vi "Close.vi"(8 "error in (no error)":errorcluster, 11 "HD44780 in":refnum<class "HD44780.lvclass">) -> (0 "error out":errorcluster)   [LabVIEW 2017, in "HD44780.lvclass"]
uses:
  HD44780.lvclass
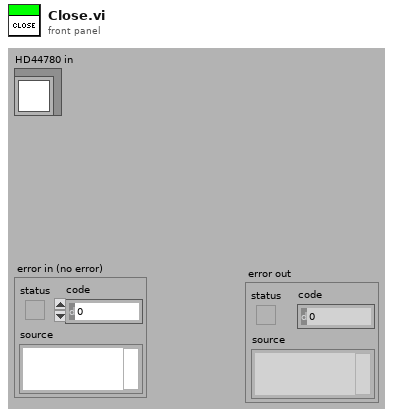
[diagram p1: front panel]
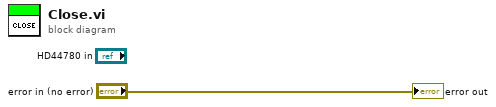
[diagram p0: block diagram]
diagram:
  "error out" <- "error in (no error)"
